vi "notifyTaskState.vi"(7 "TaskRef":refnum<vi>, 8 "error in (no error)":errorcluster, 10 "TaskRequest":T1, 11 "pdbm_taskroute_feedback_event":refnum<user-event>) -> (0 "error IO":errorcluster, 3 "pdbm_taskroute_feedback_event out":refnum<user-event>)   [LabVIEW 2015, in "pdbm_task_route.lvlib"]
uses:
  pdbm_task_route.lvlib
  UsrDefine/TaskFeedbackCmd.ctl
  pdbm_tasks/UsrDefine/TaskRequest.ctl
  pdbm_tasks/pdbm_tasks.lvlib
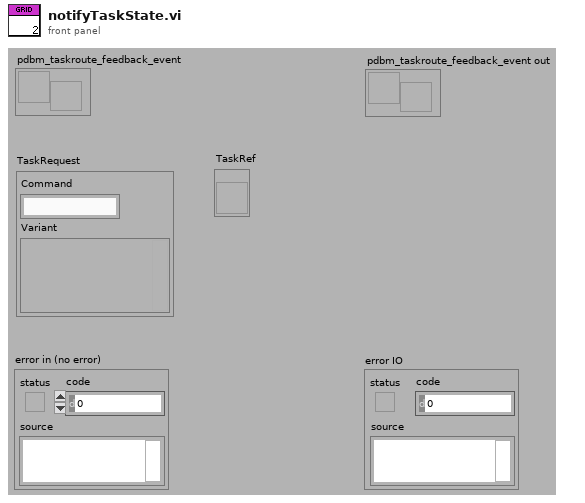
[diagram p1: front panel]
types:
  T1 = typedef "pdbm_tasks.lvlib/TaskRequest.ctl" = cluster{"Command":string, "Variant":variant}
  T2 = typedef "pdbm_task_route.lvlib/TaskFeedbackCmd.ctl" = cluster{"TaskRef":refnum<vi>, "Command":string, "Variant":variant}
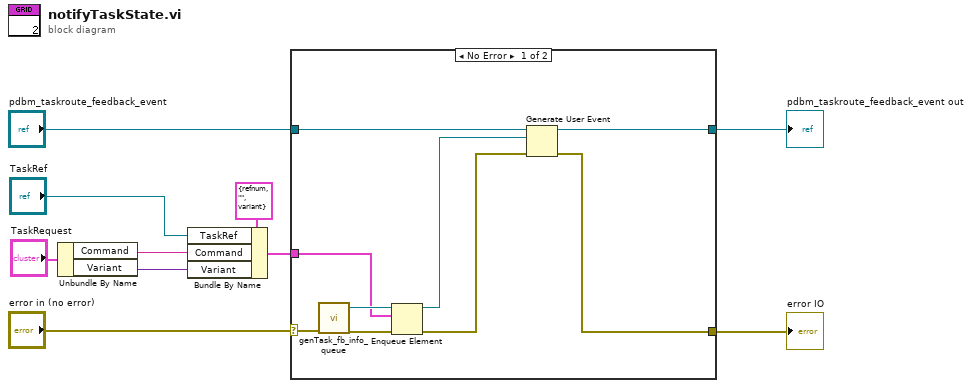
[diagram p0: block diagram]
diagram:
  n1 = Unbundle By Name("TaskRequest") -> ("Command"=w3:string, "Variant"=w2:variant)
  n2 = Bundle By Name(cluster=T2 {"TaskRef"=refnum, "Command"="", "Variant"=variant} ("element"), "TaskRef"="TaskRef", "Command"=w3, "Variant"=w2) -> (w1:T2)
  n3 = case shown="No Error" "error in (no error)" {
    selector: "error in (no error)" -> [w19 w20]
    tunnel: w1 -> [w16 _]
    tunnel: "pdbm_taskroute_feedback_event" -> [w15 w21]
    tunnel: [w11 w20] -> w7
    tunnel: [w14 w21] -> w8
    frame No Error {
      n4 = call "genTask_fb_info_queue.vi"("error in (no error)"=w19) -> ("error IO"=w17:errorcluster, "pdbm_task_fb_info_queue"=w18:refnum<queue>)  [unwired: 9 in]
      n5 = Enqueue Element(queue=w18, element=w16, error in (no error)=w17) -> (queue out=w13:refnum<queue>, error out=w12:errorcluster)  [unwired: 1 in, 1 out]
      n6 = Generate User Event(user event=w15, event data cluster=w13, error in=w12) -> (user event out=w14:refnum<user-event>, error out=w11:errorcluster)  [unwired: 1 in]
    }
    frame Error {
    }
  }
  "pdbm_taskroute_feedback_event out" <- w8
  "error IO" <- w7
